vi "calculate_bmi.vi"(11 "bmi_inputs":cluster{"weight_in_kg":dbl, "height_in_cm":dbl}={"weight_in_kg"=0.0, "height_in_cm"=2.0}) -> (3 "bmi":dbl)   [LabVIEW 2023]
panel:
  out "error out":errorcluster
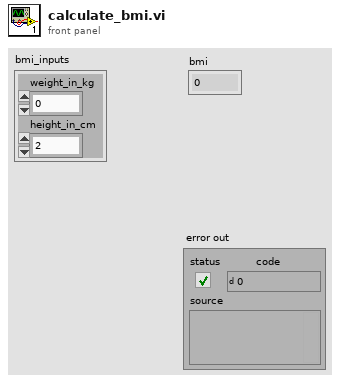
[diagram p1: front panel]
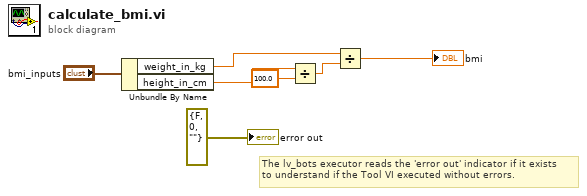
[diagram p0: block diagram]
diagram:
  # "The lv_bots executor reads the 'error out' indicator if it exists\nto understand if the Tool VI executed without errors."
  n1 = Unbundle By Name("bmi_inputs") -> ("weight_in_kg"=w3:dbl, "height_in_cm"=w6:dbl)
  n2 = Divide(x=w6, y=100.0) -> (x/y=w4:dbl)
  n3 = Divide(x=w3, y=w4) -> (x/y=→"bmi":dbl)
  "error out" <- errorcluster {"status"=FALSE, "code"=0, "source"=""} ("error out")
